vi "TCP Read.vi"() -> ()   [LabVIEW 2018]
uses:
  TCP Multiple Connections State.ctl
  Lauda Integral XT-150 TCU/TCP Library.lvlib
  support/Message Queue/Message Queue.lvlib
  support/Message Queue/Enqueue Message (Single).vi
  support/Message Queue/Message Cluster.ctl
  Main/Main Queue Cluster.ctl
  Drag and Drop/Thumbnail Cluster.ctl
  Drag and Drop/Object Type Enum.ctl
  <vilib>/Utility/miscctls.llb/LVRectTypeDef.ctl
  Drag and Drop/Object Cluster.ctl
  <vilib>/Utility/miscctls.llb/LVPositionTypeDef.ctl
  <vilib>/Utility/miscctls.llb/LVPoint32TypeDef.ctl
  TT Module/Controls/TT Module Config Cluster.ctl
  TT Module/TT Module.lvlib
  Masterflex 7550-30/Controls/Settings Cluster.ctl
  Masterflex 7550-30/Masterflex 7550-30.lvlib
  Ismatec ISM 831C/Controls/Ismatech Settings Cluster.ctl
  Ismatec ISM 831C/Ismatec ISM 831C.lvlib
  Tacmina QI/Tacmina QI DAQ Setting.ctl
  Tacmina QI/Tacmina QI.lvlib
  KNF Pump/Settings Cluster plus SIMDOS.ctl
  KNF Pump/KNF SIMDOS.lvlib
  VICI M50 Party Mode/Settings Cluster.ctl
  VICI M50 Party Mode/VICI M6 M50 Party Mode.lvlib
  FLOM Pump/Settings Cluster.ctl
  FLOM Pump/FLOM Pump.lvlib
  ASIA Pump/Pump Settings.ctl
  ASIA Pump.lvlib
  Mettler Toledo/Controls/Settings Cluster.ctl
  Mettler Toledo/Mettler Toledo.lvlib
  Bronkhorst M13 Flow Meter/Settings Cluster.ctl
  Bronkhorst M13 Flow Meter/Bronkhorst M13 Flow Meter.lvlib
  Measure Instrument/PID Input Enum.ctl
  Measure Instrument/PID 2 Output Enum.ctl
  Measure Instrument/PID 2 Parameters Cluster.ctl
  SSI PR Class/SSI PR Settings Cluster.ctl
  SSI PR Class/SSI PR Pump.lvlib
  Feed Module/Controls/Feed Module Settings Cluster.ctl
  Feed Module/Feed Module.lvlib
  Feed Module/Controls/Feed Module Config Cluster.ctl
  Acquisition/Task Cluster.ctl
  Acquisition/Hardware Configuration.ctl
  DAQ/DAQ.lvlib
  PT Module/Controls/PT Module Config Cluster.ctl
  PT Module/PT Module.lvlib
  Scale Module Folder/Feed Module/Controls/Scale Module Settings Cluster.ctl
  Scale Module Folder/Scale Module.lvlib
  Scale Module Folder/Feed Module/Controls/Scale Module Config Cluster.ctl
  Pump Module Folder/Pump Module Settings Cluster.ctl
  Pump Module Folder/Pump Module.lvlib
  Pump Module Folder/Pump Module Config Cluster.ctl
  LabJack Module/Controls/U3 Module Config Cluster.ctl
  LabJack Module/U3 Module.lvlib
  Decoration Module/Decoration Module Config Cluster.ctl
  Flow Module Folder/Feed Module/Controls/Flow Module Settings Cluster.ctl
  Flow Module Folder/Flow Module.lvlib
  Flow Module Folder/Feed Module/Controls/Flow Module Config Cluster.ctl
  TCU Module/TCU Module Folder/Measure Instrument/Output Devices.ctl
  Huber TCU/Huber Settings.ctl
  Huber TCU/Huber Ministat 230 TCU.lvlib
  Lauda Integral XT-150 TCU/Lauda Settings.ctl
  Lauda Integral XT-150 TCU/Lauda TCU.lvlib
  Julabo Type 1 TCU/Julabo Type 1 TCU Folder/Julabo FP-50 Settings.ctl
  Julabo Type 1 TCU/Julabo Type 1 TCU Folder/Julabo Type FP-50 TCU.lvlib
  Huber Unistat 410 TCU/Huber Unistat 410 Settings.ctl
  Huber Unistat 410 TCU/Huber Unistat 410 TCU.lvlib
  TCU Module/TCU Module Folder/TCU Module Settings Cluster.ctl
  TCU Module/TCU Module Folder/TCU Module.lvlib
  TCU Module/TCU Module Folder/TCU Module Config Cluster.ctl
  Sequencing/Squence Control.ctl
  Sequencing/Sequencing Library.lvlib
  D-O Module Folder/Not Sure Where this is Used.ctl
  D-O Module Folder/D-O Device Settings Cluster.ctl
  D-O Module Folder/D-O Module.lvlib
  VICI Electronic Actuator/VICI Electronic Actuator Settings.ctl
  D-O Module Folder/DIO Valve/VICI Electronic Actuator.lvlib
  D-O Module Folder/D-O Module Settings Cluster.ctl
  D-O Module Folder/Valve Clusters.ctl
  D-O Module Folder/D-O Module Config Cluster.ctl
  Pressure Transmitter/Pressure Transmitter Device Settings.ctl
  Pressure Transmitter/Pressure Transmitter Library.lvlib
  Pressure Reg Module/Pressure Regulator Device Settings.ctl
  Pressure Reg Module/Pressure Regulator Library.lvlib
  Pressure Regulator Control Module/Pressure Regulator/Controls/4-20mA Module Settings Cluster.ctl
  Pressure Regulator Control Module/Pressure Regulator/4-20mA Module.lvlib
  Pressure Regulator Control Module/Pressure Regulator/Controls/4-20mA Module Config Cluster.ctl
  OPC/OPC Settings.ctl
  OPC/OPC UA.lvlib
  <vilib>/OPCUA/controls/NodeId.ctl
  <vilib>/OPCUA/controls/OPC UA StatusCode.ctl
  OPC/Variable Data Cluster.ctl
  Scale Module Folder/Measure Instrument/State Enum.ctl
  Scale Module Folder/Measure Instrument/Scale Module Engine.lvlib
  <vilib>/OPCUA/controls/Subscription ID.ctl
  <vilib>/OPCUA/controls/OPC UA Client Refnum.ctl
  <vilib>/OPCUA/controls/Data Type.ctl
  <vilib>/OPCUA/controls/Subscription Data Change.ctl
  OPC/OPC Module Config.ctl
  Config Module/Controls/Main Config Cluster.ctl
  Config Module/Config Module.lvlib
  Drag and Drop/State Cluster.ctl
  Drag and Drop/Drag and Drop.lvlib
panel:
  in  "Input":T1 {"Main Config"."PR Module Configs"."Settings"."PID 2 Parameters"."output range"."output low" format="%.2f"; "Main Config"."PR Module Configs"."Settings"."PID 2 Parameters"."output range"."output high" min=0.0 max=100.0 format="%.2f"; "Main Config"."PR Module Configs"."Settings"."PID 2 Parameters"."PID gains"."derivative time (Td, min)" format="%.3f"; "Main Config"."PR Module Configs"."Settings"."PID 2 Parameters"."PID gains"."integral time (Ti, min)" format="%.3f"; "Main Config"."PR Module Configs"."Settings"."PID 2 Parameters"."PID gains"."proportional gain (Kc)" format="%.3f"; "Main Config"."Steps"."Control" items=["Pump %", "Setpoint"]; "Main Config"."TCU Module Configs"."Settings"."Julabo FP-50 Settings"."Pump Power" min=0 max=8 step=1; "Main Config"."TCU Module Configs"."Settings"."Lauda Settings"."Pump Power" min=0 max=8 step=1; "Main Config"."Pump Module Configs"."Settings"."ASIA Pump C"."channel" min=0 max=1 step=1; "Main Config"."Pump Module Configs"."Settings"."Masterflex"."Pump Number" min=1.0 max=20.0 step=1.0; "Main Config"."Pump Module Configs"."Settings"."Ismatech"."Pump Number" min=1.0 max=20.0 step=1.0; "Main Config"."Feed Module Configs"."Settings"."output range"."output low" min=0.0 max=100.0 format="%.2f"; "Main Config"."Feed Module Configs"."Settings"."output range"."output high" format="%.2f"; "Main Config"."Feed Module Configs"."Settings"."PID 2 Parameters"."PID gains"."derivative time (Td, min)" format="%.3f"; "Main Config"."Feed Module Configs"."Settings"."PID 2 Parameters"."PID gains"."integral time (Ti, min)" format="%.3f"; "Main Config"."Feed Module Configs"."Settings"."PID 2 Parameters"."PID gains"."proportional gain (Kc)" format="%.3f"; "Main Config"."Feed Module Configs"."Settings"."ASIA Pump C"."channel" min=0 max=1 step=1; "Main Config"."Feed Module Configs"."Settings"."Ismatech"."Pump Number" min=1.0 max=20.0 step=1.0; "Main Config"."Feed Module Configs"."Settings"."Masterflex"."Pump Number" min=1.0 max=20.0 step=1.0}
  in  "error in (no error)":errorcluster
  in  "address":string="10.131.72.83"
  in  "port":u16=50023
  in  "Message Queues out":T62
  # "Instrument Settings"
  # "Instrument Settings"
  # "Output Instruments"
  # "Flow Meter Settings"
  # "Output Instruments"
  # "Scale Settings"
  # "Output Instruments"
  # "Input Instruments"
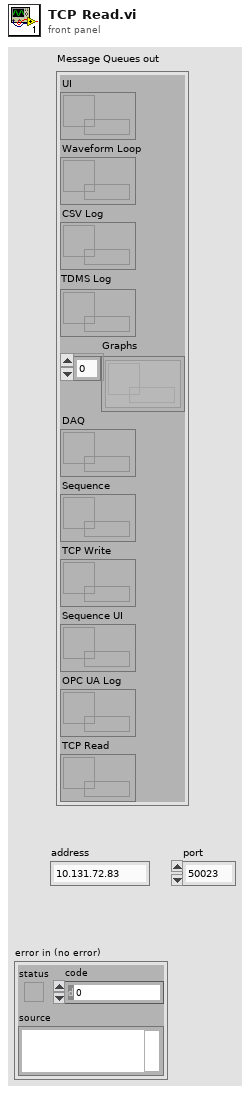
[diagram p1: front panel]
types:
  T1 = typedef "Drag and Drop.lvlib/State Cluster.ctl" = cluster{"VI refs":refnum<vi>[], "Queues":refnum<queue>[], "[Thumbnails]":T2[], "Drag Object Idx":i32, "[Objects]":T3[], "Active Object":i32, "Drop Offset":T6, "Process Name":string, "Main Config":T7, "Campaign Filepath":path, "Config Changed?":bool}
  T2 = typedef "Thumbnail Cluster.ctl" = cluster{"Path":path, "Rectangle":cluster{"left":i16, "top":i16, "right":i16, "bottom":i16}}
  T3 = typedef "Object Cluster.ctl" = cluster{"BMP Path":path, "Anchor Position":cluster{"X":i32, "Y":i32}, "Hot Spot":T4, "Type":T5, "Parameters":variant}
  T4 = typedef "LVRectTypeDef.ctl" = cluster{"Left":i16, "Top":i16, "Right":i16, "Bottom":i16}
  T5 = typedef "Object Type Enum.ctl" = enum16{"Icon", "Line", "Text", "Feed Module"}
  T6 = typedef "LVPositionTypeDef.ctl" = cluster{"Left":i32, "Top":i32}
  T7 = typedef "Config Module.lvlib/Main Config Cluster.ctl" = cluster{"OPC Module Configs":T8[], "Feed Module Configs":T17[], "Log File Path":path, "TT Module Configs":T32[], "DAQ Config":T33, "PT Module Configs":T35[], "Scale Module Configs":T36[], "Pump Module Configs":T38[], "U3 Module Configs":T40[], "Decoration Module Configs":T41[], "Flow Module Configs":T42[], "TCU Module Configs":T44[], "Steps":T51, "Abort":bool, "DO Module Configs":T53[], "PR Module Configs":T58[], "Cycle Period":dbl}
  T8 = typedef "OPC UA.lvlib/OPC Module Config.ctl" = cluster{"State":T9, "GUID":string, "Drop Coords":T10, "Configuration":T11, "First Iteration":bool, "Data":cluster{"Object Name":string, "Variable Array":T12[]}[], "Process Name":string, "Load Count":i32, "Log Started":bool, "subscription ID out":T15, "OPC UA client refnum out":T16, "Event Registration Refnum":refnum<event-registration>, "Start Time":timestamp, "Current Time":timestamp}
  T9 = typedef "Scale Module.lvlib/Scale Module Engine.lvlib/State Enum.ctl" = enum16{"Measuring", "Idle"}
  T10 = typedef "LVPoint32TypeDef.ctl" = cluster{"Horizontal":i32, "Vertical":i32}
  T11 = typedef "OPC UA.lvlib/OPC Settings.ctl" = cluster{"Cycle Period":dbl, "server endpoint URL":string, "security policy":cluster{"message mode":enum16{"None", "Sign", "Sign and Encrypt"}, "security":enum16{"Basic256", "Basic128Rsa15"}}, "Trust Any Server":bool}
  T12 = typedef "OPC UA.lvlib/Variable Data Cluster.ctl" = cluster{"node ID":T13, "browse name":string, "status":T14, "timestamp":timestamp, "value ":variant}
  T13 = typedef "NodeId.ctl" = string
  T14 = typedef "OPC UA StatusCode.ctl" = u32
  T15 = typedef "Subscription ID.ctl" = u32
  T16 = typedef "OPC UA Client Refnum.ctl" = refnum<k21>
  T17 = typedef "Feed Module.lvlib/Feed Module Config Cluster.ctl" = cluster{"GUID":string, "Drop Coords":T10, "Process Name":string, "Queue Name":string, "Settings":T18, "Settings Load Count":i32, "OP Load Count":i32}
  T18 = typedef "Feed Module.lvlib/Feed Module Settings Cluster.ctl" = cluster{"Cycle Period":dbl, "Ismatech":T19, "Masterflex":T20, "Mettler":T21, "Bronkhorst M13 Flow Meter":T22, "PID 2 Parameters":T23, "Manual Entry":dbl, "Auto?":bool, "output range":cluster{"output high":dbl, "output low":dbl}, "Bronkhorst M14":T21, "Tacmina Settings":T26, "KNF SIMDOS Settings":T27, "ASIA Pump C":T28, "VICI Settings":T29, "FLOM Settings":T30, "SSI PR Settings":T31}
  T19 = typedef "Ismatec ISM 831C.lvlib/Ismatech Settings Cluster.ctl" = cluster{"VISA resource name":refnum<visa-resource-name>, "Simulated?":bool, "Pump Number":dbl, "Reverse?":bool}
  T20 = typedef "Masterflex 7550-30.lvlib/Settings Cluster.ctl" = cluster{"VISA resource name":refnum<visa-resource-name>, "Simulated?":bool, "Pump Number":dbl, "Reverse?":bool}
  T21 = typedef "Mettler Toledo.lvlib/Settings Cluster.ctl" = cluster{"VISA resource name":refnum<visa-resource-name>, "Simulated?":bool}
  T22 = typedef "Bronkhorst M13 Flow Meter.lvlib/Settings Cluster.ctl" = cluster{"VISA resource name":refnum<visa-resource-name>, "Simulated?":bool}
  T23 = typedef "PID 2 Parameters Cluster.ctl" = cluster{"Input Device":T24, "Output Device":T25, "Setpoint":dbl, "PID gains":cluster{"proportional gain (Kc)":dbl, "integral time (Ti, min)":dbl, "derivative time (Td, min)":dbl}}
  T24 = typedef "PID Input Enum.ctl" = enum16{"Default", "Bronkhorst M13", "Bronkhorst M14", "Scale Rate of Change"}
  T25 = typedef "PID 2 Output Enum.ctl" = enum16{"Default", "Ismatec ISM 831C", "Masterflex 7550-30", "VICI", "Tacmina QI", "KNF SIMDOS", "ASIA Type C", "FLOM UI-22-11", "SSI PR"}
  T26 = typedef "Tacmina QI.lvlib/Tacmina QI DAQ Setting.ctl" = cluster{"Analog DAQ Task":refnum<k21>, "Digital DAQ Task":refnum<k21>}
  T27 = typedef "KNF SIMDOS.lvlib/Settings Cluster plus SIMDOS.ctl" = cluster{"VISA resource name":refnum<visa-resource-name>, "Simulated?":bool}
  T28 = typedef "ASIA Pump.lvlib/Pump Settings.ctl" = cluster{"ASIA Pump #":i32, "channel":i32, "Simulated":bool}
  T29 = typedef "VICI M6 M50 Party Mode.lvlib/Settings Cluster.ctl" = cluster{"VISA resource name":refnum<visa-resource-name>, "Simulated?":bool, "Pump Letter":string, "Reverse?":bool}
  T30 = typedef "FLOM Pump.lvlib/Settings Cluster.ctl" = cluster{"VISA resource name":refnum<visa-resource-name>, "Simulated?":bool, "Pump Number":dbl}
  T31 = typedef "SSI PR Pump.lvlib/SSI PR Settings Cluster.ctl" = cluster{"VISA resource name":refnum<visa-resource-name>, "Simulated?":bool}
  T32 = typedef "TT Module.lvlib/TT Module Config Cluster.ctl" = cluster{"GUID":string, "Drop Coords":T10, "Input Channel Tag Name ":string, "Process Name":string, "Queue Name":string, "Input Channel Numeric Alarm Settings":cluster{"enable? (F)":bool, "name":string, "alarm type":enum16{"HI_HI", "HI", "LO", "LO_LO"}, "level/change":dbl, "deadband/time":dbl, "priority":u32, "ack type":enum16{"Auto", "User", "None", "Each Occurrence"}, "area":string, "description":string, "log? (T)":bool}[]}
  T33 = typedef "DAQ.lvlib/Hardware Configuration.ctl" = cluster{"Tasks":T34[]}
  T34 = typedef "Task Cluster.ctl" = cluster{"DAQmx Task":refnum<k21>, "Read-Write Radio":enum32{"Read", "Write"}}
  T35 = typedef "PT Module.lvlib/PT Module Config Cluster.ctl" = cluster{"GUID":string, "Drop Coords":T10, "Input Channel Tag Name ":string, "Process Name":string, "Queue Name":string, "Input Channel Numeric Alarm Settings":cluster{"enable? (F)":bool, "name":string, "alarm type":enum16{"HI_HI", "HI", "LO", "LO_LO"}, "level/change":dbl, "deadband/time":dbl, "priority":u32, "ack type":enum16{"Auto", "User", "None", "Each Occurrence"}, "area":string, "description":string, "log? (T)":bool}[]}
  T36 = typedef "Scale Module.lvlib/Scale Module Config Cluster.ctl" = cluster{"GUID":string, "Drop Coords":T10, "Process Name":string, "Queue Name":string, "Settings":T37, "Load Count":i32}
  T37 = typedef "Scale Module.lvlib/Scale Module Settings Cluster.ctl" = cluster{"Cycle Period":dbl, "Mettler":T21, "Scale Type":string}
  T38 = typedef "Pump Module.lvlib/Pump Module Config Cluster.ctl" = cluster{"GUID":string, "Drop Coords":T10, "Process Name":string, "Queue Name":string, "Settings":T39, "Load Count":i32}
  T39 = typedef "Pump Module.lvlib/Pump Module Settings Cluster.ctl" = cluster{"Cycle Period":dbl, "Ismatech":T19, "Masterflex":T20, "Manual Entry":dbl, "VICI Settings":T29, "Output Device":T25, "Tacmina Settings":T26, "KNF SIMDOS Settings":T27, "ASIA Pump C":T28, "FLOM Settings":T30, "Pump Calibration File":path, "Calibration":dbl, "Pump Cal Enum":u16, "SSI PR Settings":T31}
  T40 = typedef "U3 Module.lvlib/U3 Module Config Cluster.ctl" = cluster{"GUID":string, "Drop Coords":T10, "AI Channel Number":enum16{"Default", "AI0", "AI1", "AI2", "AI3", "AI4", "AI5", "AI6", "AI7"}, "Process Name":string, "Queue Name":string, "Input Channel Numeric Alarm Settings":cluster{"enable? (F)":bool, "name":string, "alarm type":enum16{"HI_HI", "HI", "LO", "LO_LO"}, "level/change":dbl, "deadband/time":dbl, "priority":u32, "ack type":enum16{"Auto", "User", "None", "Each Occurrence"}, "area":string, "description":string, "log? (T)":bool}[]}
  T41 = typedef "Decoration Module Config Cluster.ctl" = cluster{"GUID":string, "Drop Coords":T10, "Decoration Filepath":path}
  T42 = typedef "Flow Module.lvlib/Flow Module Config Cluster.ctl" = cluster{"GUID":string, "Drop Coords":T10, "Process Name":string, "Queue Name":string, "Settings":T43, "Load Count":i32}
  T43 = typedef "Flow Module.lvlib/Flow Module Settings Cluster.ctl" = cluster{"Cycle Period":dbl, "Bronkhorst M13":T21, "Flow Meter Type":string, "Bronkhorst M14":T21}
  T44 = typedef "TCU Module.lvlib/TCU Module Config Cluster.ctl" = cluster{"GUID":string, "Drop Coords":T10, "Process Name":string, "Queue Name":string, "Settings":T45, "Load Count":i32, "Power Level Changed":bool}
  T45 = typedef "TCU Module.lvlib/TCU Module Settings Cluster.ctl" = cluster{"Cycle Period":dbl, "Setpoint Entry":dbl, "Output Device":T46, "Huber Ministat 230 Settings":T47, "Lauda Settings":T48, "Julabo FP-50 Settings":T49, "Internal Control?":bool, "Huber Unistat 410 Settings":T50}
  T46 = typedef "Output Devices.ctl" = enum16{"Default", "Huber Ministat 230", "Huber Unistat 410", "Lauda XT-150", "Julabo FP-50"}
  T47 = typedef "Huber Ministat 230 TCU.lvlib/Huber Settings.ctl" = cluster{"VISA resource name":refnum<visa-resource-name>, "Simulated?":bool}
  T48 = typedef "Lauda TCU.lvlib/Lauda Settings.ctl" = cluster{"VISA resource name":refnum<visa-resource-name>, "Simulated?":bool, "Pump Power":i32}
  T49 = typedef "Julabo Type FP-50 TCU.lvlib/Julabo FP-50 Settings.ctl" = cluster{"VISA resource name":refnum<visa-resource-name>, "Simulated?":bool, "Pump Power":i32}
  T50 = typedef "Huber Unistat 410 TCU.lvlib/Huber Unistat 410 Settings.ctl" = cluster{"VISA resource name":refnum<visa-resource-name>, "Simulated?":bool}
  T51 = typedef "Not Sure Where this is Used.ctl" = T52[]
  T52 = typedef "Sequencing Library.lvlib/Squence Control.ctl" = cluster{"Module":string, "Control":u16, "Value":dbl, "Wait (sec)":dbl}
  T53 = typedef "D-O Module.lvlib/D-O Module Config Cluster.ctl" = cluster{"GUID":string, "Drop Coords":T10, "Process Name":string, "Queue Name":string, "Settings":T54, "Load Count":i32}
  T54 = typedef "D-O Module.lvlib/Valve Clusters.ctl" = cluster{"Valve Settings":T55, "Valve Type":enum16{"Default", "Digital Output Valve", "VICI Electronic Actuator"}, "Time On (Sec)":dbl, "Time Off (Sec)":dbl, "Run?":bool}
  T55 = typedef "D-O Module.lvlib/D-O Module Settings Cluster.ctl" = cluster{"D-O Settings":T56, "VICI Electronic Actuator":T57}
  T56 = typedef "D-O Module.lvlib/D-O Device Settings Cluster.ctl" = cluster{"DAQmx Task Name":refnum<k21>, "Output Channel":u16, "Output Channel Names":string[]}
  T57 = typedef "VICI Electronic Actuator.lvlib/VICI Electronic Actuator Settings.ctl" = cluster{"VISA resource name":refnum<visa-resource-name>, "Mode":enum16{"Two Positions With Stops", "Two Positions Without Stops", "Mutiposition"}, "Simulated":bool}
  T58 = typedef "4-20mA Module.lvlib/4-20mA Module Config Cluster.ctl" = cluster{"GUID":string, "Drop Coords":T10, "Process Name":string, "Queue Name":string, "Settings":T59, "Settings Load Count":i32}
  T59 = typedef "4-20mA Module.lvlib/4-20mA Module Settings Cluster.ctl" = cluster{"Cycle Period":dbl, "PID 2 Parameters":cluster{"Input Device":enum16{"Default", "4-20mA"}, "Output Device":enum16{"Default", "Equilibar Pressure Reg", "Flow Regulator"}, "Setpoint":dbl, "PID gains":cluster{"proportional gain (Kc)":dbl, "integral time (Ti, min)":dbl, "derivative time (Td, min)":dbl}, "output range":cluster{"output low":dbl, "output high":dbl}}, "Manual Entry":dbl, "Auto?":bool, "4-20mA Input Settings":T60, "4-20mA Out Settings":T61, "Input Channel Tag Name ":string}
  T60 = typedef "Pressure Transmitter Library.lvlib/Pressure Transmitter Device Settings.ctl" = cluster{"Input Channel ":u16}
  T61 = typedef "Pressure Regulator Library.lvlib/Pressure Regulator Device Settings.ctl" = cluster{"Output DAQ Task":refnum<k21>}
  T62 = typedef "Main Queue Cluster.ctl" = cluster{"UI":refnum<queue>, "Waveform Loop":refnum<queue>, "CSV Log":refnum<queue>, "TDMS Log":refnum<queue>, "Graphs":refnum<queue>[], "DAQ":refnum<queue>, "Sequence":refnum<queue>, "TCP Write":refnum<queue>, "Sequence UI":refnum<queue>, "OPC UA Log":refnum<queue>, "TCP Read":refnum<queue>}
  T63 = typedef "TCP Library.lvlib/TCP Multiple Connections State.ctl" = enum16{"Initialize", "Status Check", "Send Data", "Stop"}
  T64 = cluster{"listener ID":refnum<k5>, "State":T63, "Clients":refnum<k5>[], "ELN Number":string}
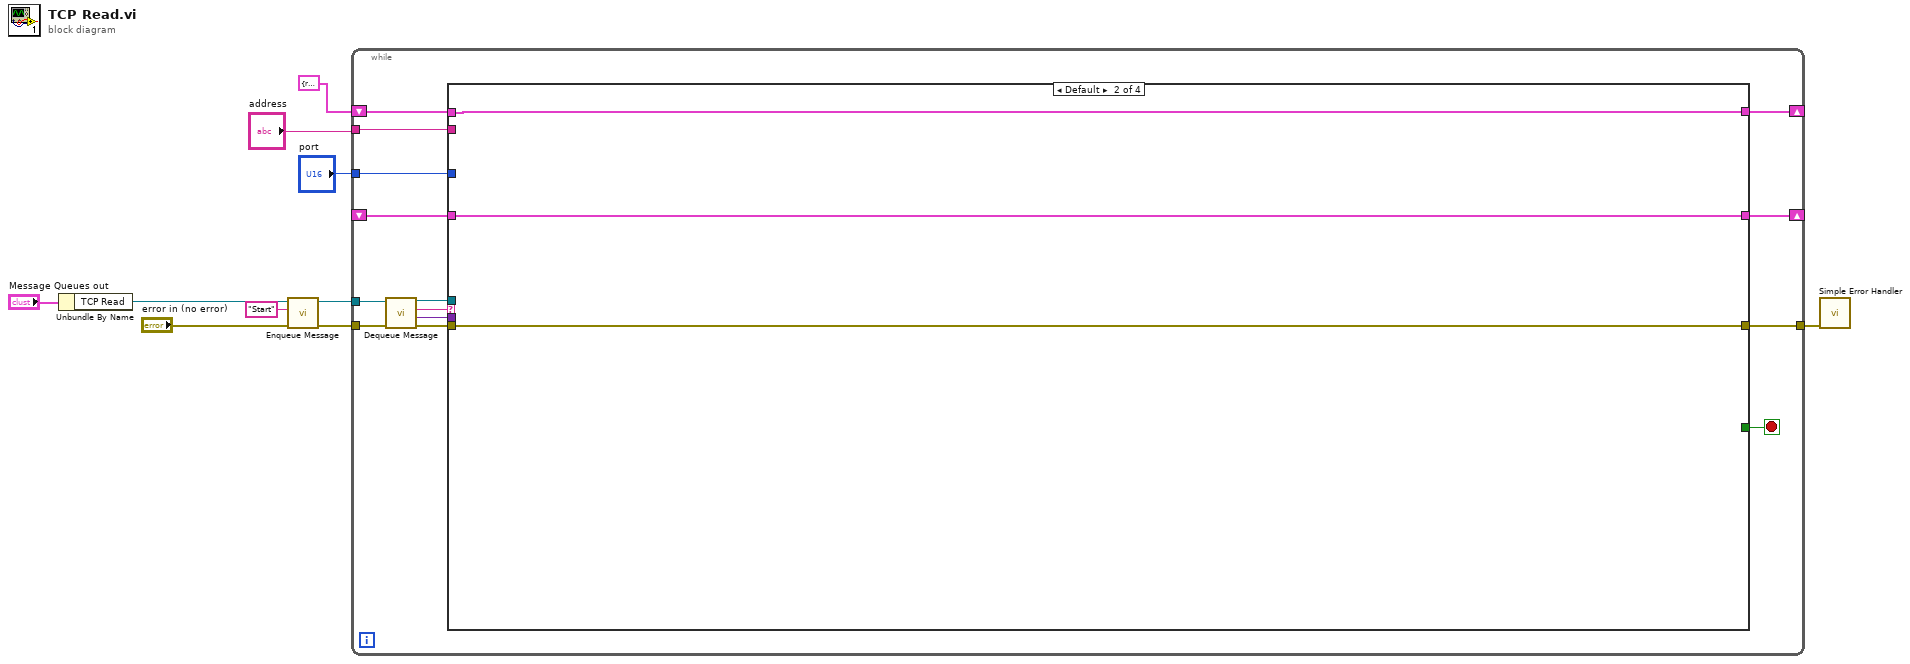
[diagram p0: block diagram]
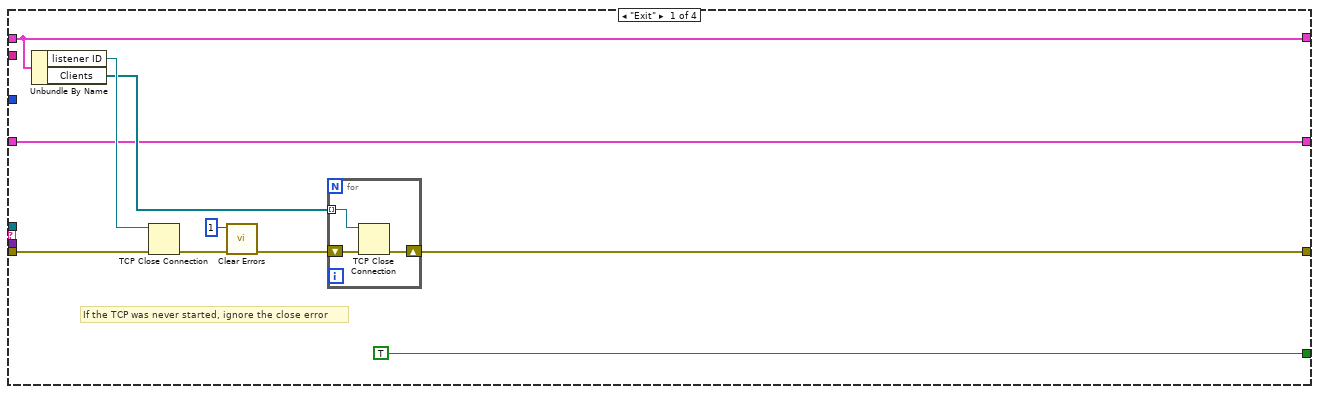
[diagram p2: hidden frame]
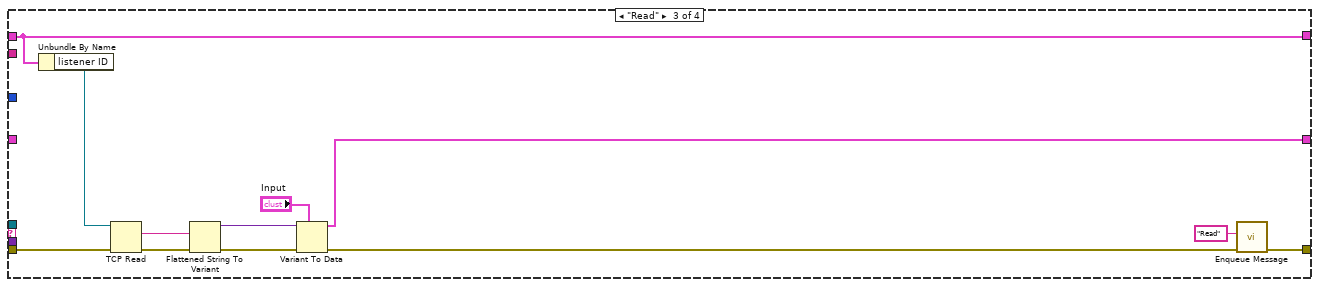
[diagram p3: hidden frame]
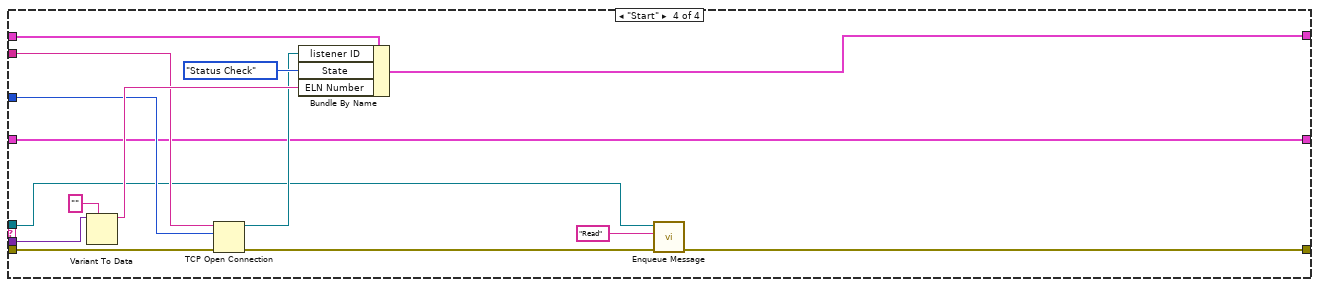
[diagram p4: hidden frame]
diagram:
  n1 = Unbundle By Name("Message Queues out") -> ("TCP Read"=w4:refnum<queue>)
  n2 = call-poly "Enqueue Message.vi"("error in (no error)"="error in (no error)", "Message"="Start", "Message Queue"=w4) -> ("error out"=w2:errorcluster, "dup Message Queue"=w1:refnum<queue>)  [unwired: 7 in]
  n3 = while {
    tunnel: w1 -> [w22]
    shift-right: [w19] -> _
    shift-left: T64 {"listener ID"=refnum, "State"=enum."Initialize", "Clients"=[], "ELN Number"=""} -> [w18]
    tunnel: [w17] -> w8
    tunnel: "port" -> [w16]
    tunnel: "address" -> [w15]
    tunnel: w2 -> [w14]
    shift-right: [w12] -> _
    shift-left: _ -> [w11]
    stop <- w21 stop-if-true
    n4 = call "Dequeue Message.vi"("error in (no error)"=w14, "Message Queue"=w22) -> ("error out"=w23:errorcluster, "Message Data"=w20:variant, "Message"=w24:string, "dup Message Queue"=w13:refnum<queue>)  [unwired: 6 in]
    n5 = case shown="Default" w24 {
      tunnel: w23 -> [w34 w39 w50 w58]
      tunnel: [TRUE _ _ _] -> w21
      tunnel: w20 -> [_ _ _ w64]
      tunnel: [w29 w40 w49 w66] -> w19
      tunnel: w18 -> [w29 w40 w49 w67]
      tunnel: [w30 w39 w51 w55] -> w17
      tunnel: w16 -> [_ _ _ w60]
      tunnel: w15 -> [_ _ _ w59]
      tunnel: w13 -> [_ _ _ w54]
      tunnel: [w25 w38 w41 w53] -> w12
      tunnel: w11 -> [w25 w38 _ w53]
      frame "Exit" {
        # "If the TCP was never started, ignore the close error"
        n6 = Unbundle By Name(w29) -> ("listener ID"=w32:refnum<k5>, "Clients"=w31:refnum<k5>[])
        n7 = TCP Close Connection(connection ID=w32, error in (no error)=w34) -> (error out=w28:errorcluster)  [unwired: 1 in, 1 out]
        n8 = call <vilib>:"Clear Errors.vi"("error in (no error)"=w28, "specific error code to clear (0: all)"=1) -> ("error out"=w27:errorcluster)  [unwired: 4 in, 1 out]
        n9 = for {
          shift-right: [w36] -> w30
          shift-left: w27 -> [w37]
          tunnel: w31 -> [w35] mode=indexing
          n10 = TCP Close Connection(connection ID=w35, error in (no error)=w37) -> (error out=w36:errorcluster)  [unwired: 1 in, 1 out]
        }
      }
      frame Default {
      }
      frame "Read" {
        n11 = Unbundle By Name(w49) -> ("listener ID"=w48:refnum<k5>)
        n12 = TCP Read(connection ID=w48, error in (no error)=w50) -> (data out=w45:string, error out=w43:errorcluster)  [unwired: 3 in, 1 out]
        n13 = Flattened String To Variant(4:w43, 6:w45) -> (0:w42:errorcluster, 3:w44:variant)  [unwired: 1 in]
        n14 = Variant To Data(error in=w42, type="Input", Variant=w44) -> (data=w41:T1, error out=w46:errorcluster)
        n15 = call-poly "Enqueue Message.vi"("error in (no error)"=w46, "Message"="Read") -> ("error out"=w51:errorcluster)  [unwired: 8 in, 1 out]
      }
      frame "Start" {
        n16 = Variant To Data(type="", Variant=w64) -> (data=w62:string)  [unwired: 1 in, 1 out]
        n17 = TCP Open Connection(address=w59, remote port or service name=w60, error in (no error)=w58) -> (connection ID=w61:refnum<k5>, error out=w56:errorcluster)  [unwired: 2 in]
        n18 = Bundle By Name(cluster=w67, "listener ID"=w61, "State"=TCP_Multiple_Connections_State."Status Check" ("Initial State"), "ELN Number"=w62) -> (w66:T64)
        n19 = call-poly "Enqueue Message.vi"("error in (no error)"=w56, "Message"="Read", "Message Queue"=w54) -> ("error out"=w55:errorcluster)  [unwired: 7 in, 1 out]
      }
    }
  }
  n20 = call <vilib>:"Simple Error Handler.vi"("error in (no error)"=w8) -> ()  [unwired: 4 in, 5 out]
